vi "Validate Control Packet.vi"(11 "Control Packet":u8[](array[numeric]) format="%08b") -> (0 "Payload":u8[](array[numeric]) format="%08b", 1 "Packet Identifier":u16 format="%016b", 2 "Valid":bool, 3 "Control Packet Type":T1)   [LabVIEW 2013]
uses:
  Control Packet Type -- enum.ctl
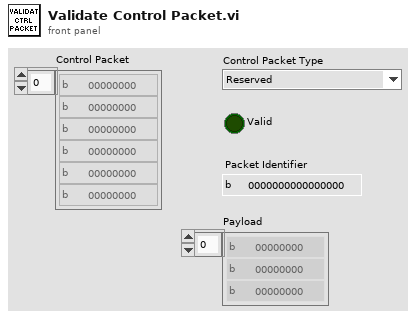
[diagram p1: front panel]
types:
  T1 = typedef "Control Packet Type -- enum.ctl" = enum16{"Reserved", "CONNECT", "CONNACK", "PUBLISH", "PUBACK", "PUBREC", "PUBREL", "PUBCOMP", "SUBSCRIBE", "SUBACK", "UNSUBSCRIBE", "UNSUBACK", "PINGREQ", "PINGRESP", "DISCONNECT", "Reserved(15)"}
  T2 = typedef "QualityOfService -- enum.ctl" = enum16{"0 (At Most Once)", "1 (At Least Once)", "2 (Exactly Once)"}
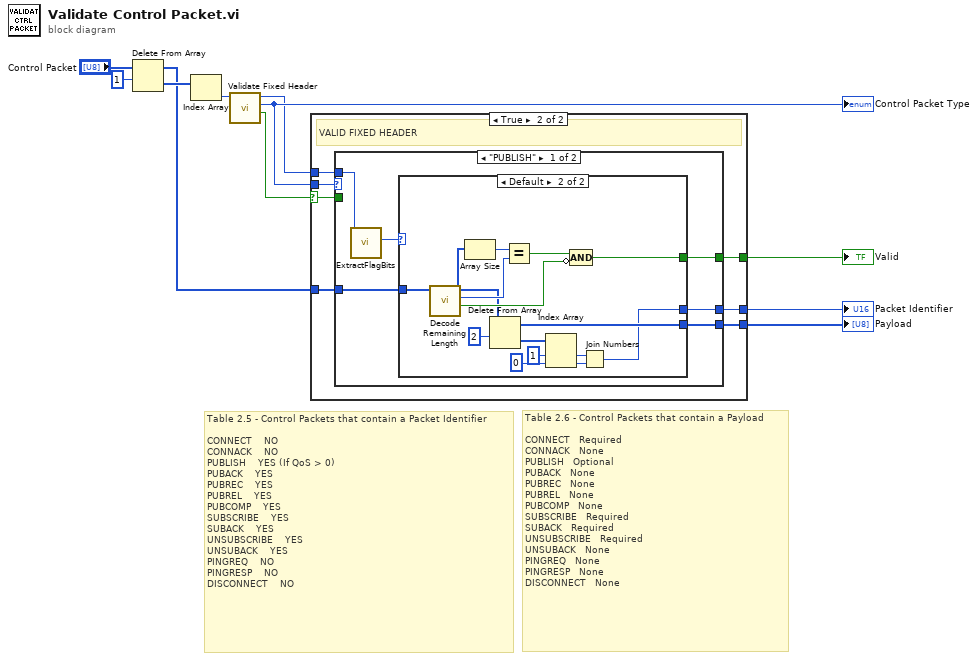
[diagram p0: block diagram]
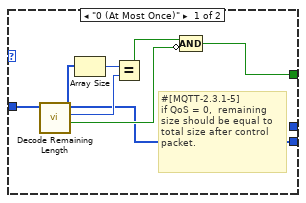
[diagram p3: hidden frame]
diagram:
  # "Table 2.5 - Control Packets that contain a Packet Identifier\n\nCONNECT    NO\nCONNACK    NO\nPUBLISH    YES (If QoS > 0)\nPUBACK    YES\nPUBREC    YES\nPUBREL    YES\nPUBCOMP    YES\nSUBSCRIBE    YES\nSUBACK    YES\nUNSUBSCRIBE    YES\nUNSUBACK    YES\nPINGREQ    NO\nPINGRESP    NO\nDISCONNECT    NO"
  # "Table 2.6 - Control Packets that contain a Payload\n\nCONNECT   Required\nCONNACK   None\nPUBLISH   Optional\nPUBACK   None\nPUBREC   None\nPUBREL   None\nPUBCOMP   None\nSUBSCRIBE   Required\nSUBACK   Required\nUNSUBSCRIBE   Required\nUNSUBACK   None\nPINGREQ   None\nPINGRESP   None\nDISCONNECT   None"
  n1 = Delete From Array(array="Control Packet", length=1) -> (deleted portion=w3:u8[], array with subset deleted=w1:u8[])  [unwired: 1 in]
  n2 = Index Array(array=w3) -> (element=w11:u8)  [unwired: 1 in]
  n3 = call "Validate Fixed Header.vi"("Fixed Header"=w11) -> ("Valid"=w7:bool, "Control Packet Type"=w9:T1, "Fixed Header dup"=w8:u8)  [unwired: 8 in]
  "Control Packet Type" <- w9
  n4 = case shown="True" w7 {
    selector: w7 -> [_ w16]
    tunnel: w1 -> [_ w18]
    tunnel: w9 -> [_ w17]
    tunnel: [_ w15] -> w10
    tunnel: w8 -> [_ w14]
    tunnel: [_ w13] -> w6
    tunnel: [_ w12] -> w5
    frame False {
      # "INVALID FIXED HEADER"
    }
    frame True {
      # "VALID FIXED HEADER"
      n5 = case shown="\"PUBLISH\"" w17 {
        tunnel: w18 -> [w24 _]
        tunnel: w16 -> [_ _]
        tunnel: [w21 _] -> w15
        tunnel: w14 -> [w23 _]
        tunnel: [w20 _] -> w13
        tunnel: [w19 _] -> w12
        frame "PUBLISH" {
          n6 = call "ExtractFlagBits.vi"("Fixed Header"=w23) -> ("QoS"=w22:T2)  [unwired: 7 in, 3 out]
          n7 = case shown="Default" w22 {
            tunnel: w24 -> [w31 w46]
            tunnel: [w26 w41] -> w21
            tunnel: [_ w34] -> w20
            tunnel: [w25 w38] -> w19
            frame "0 (At Most Once)" {
              # "#[MQTT-2.3.1-5]\nif QoS = 0,  remaining size should be equal to total size after control packet."
              n8 = call "Decode Remaining Length.vi"("Packets without 1st byte"=w31) -> ("Malformed Remaining Length"=w28:bool, "Remaining Length (bytes)"=w30:u32, "Remaining Packets"=w25:u8[])  [unwired: 8 in]
              n9 = Array Size(array=w25) -> (size(s)=w29:i32)
              n10 = Equal?(x=w29, y=w30) -> (x = y?=w27:bool)
              n11 = Compound Arithmetic op=AND(w27, invert w28) -> (w26:bool)
            }
            frame Default {
              n12 = call "Decode Remaining Length.vi"("Packets without 1st byte"=w46) -> ("Malformed Remaining Length"=w43:bool, "Remaining Length (bytes)"=w45:u32, "Remaining Packets"=w40:u8[])  [unwired: 8 in]
              n13 = Array Size(array=w40) -> (size(s)=w44:i32)
              n14 = Delete From Array(array=w40, length=2) -> (deleted portion=w37:u8[], array with subset deleted=w38:u8[])  [unwired: 1 in]
              n15 = Equal?(x=w44, y=w45) -> (x = y?=w42:bool)
              n16 = Index Array(array=w37, index #1=1 ("index"), index #2=0 ("index")) -> (element #1=w35:u8, element #2=w36:u8)
              n17 = Compound Arithmetic op=AND(w42, invert w43) -> (w41:bool)
              n18 = Join Numbers(hi=w35, lo=w36) -> ((hi.lo)=w34:u16)
            }
          }
        }
        frame "CONNECT" {
        }
      }
    }
  }
  "Valid" <- w10
  "Packet Identifier" <- w6
  "Payload" <- w5
